vi "chooseSignal.vi"(7 "countIN":dbl, 8 "Direction":string, 9 "signalIN":dbl[](array[numeric]), 10 "chosen?":bool, 11 "Path":string) -> (1 "signalOUT":dbl[](array[numeric]), 6 "countOUT":dbl)   [LabVIEW 2019]
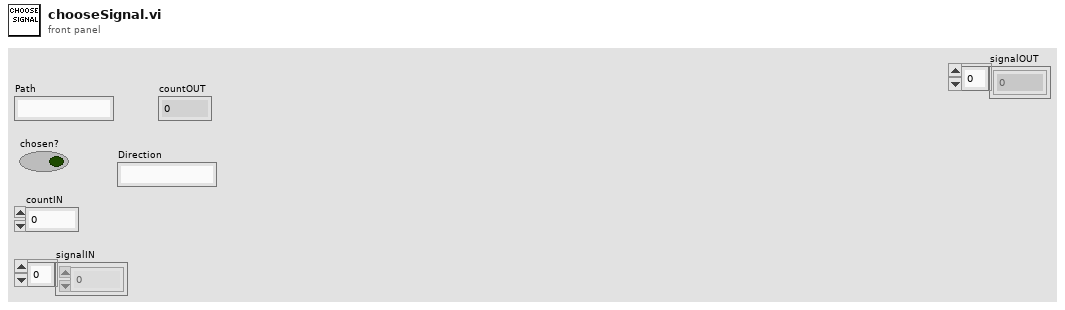
[diagram p1: front panel]
types:
  T1 = enum16{"open", "replace", "create", "open or create", "replace or create", "replace or create with confirmation"}
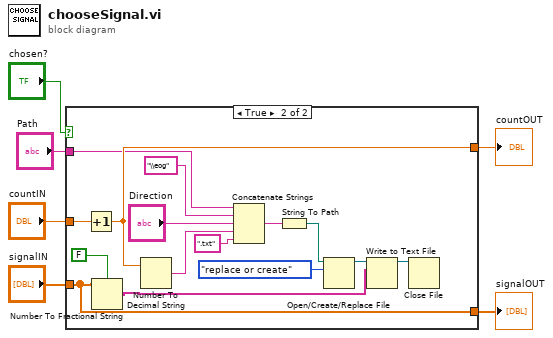
[diagram p0: block diagram]
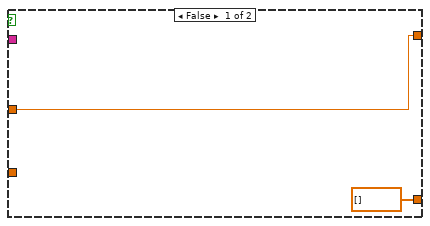
[diagram p2: hidden frame]
diagram:
  n1 = case shown="True" "chosen?" {
    tunnel: "countIN" -> [w8 w23]
    tunnel: [w8 w22] -> w3
    tunnel: [dbl[] [] ("pico -") w10] -> w1
    tunnel: "Path" -> [_ w14]
    tunnel: "signalIN" -> [_ w10]
    frame False {
    }
    frame True {
      n2 = Increment(x=w23) -> (x+1=w22:dbl)
      n3 = Number To Fractional String(use system decimal point (T)=FALSE, number=w10) -> (F-format string=w11:string[])  [unwired: 2 in]
      n4 = Number To Decimal String(number=w22) -> (decimal integer string=w21:string)  [unwired: 1 in]
      n5 = Concatenate Strings(w14, "\\eog" ("string"), "Direction", w21, ".txt" ("string")) -> (w19:string)
      n6 = String To Path(string=w19) -> (path=w18:path)
      n7 = Open/Create/Replace File(file path (use dialog)=w18, operation (0:open)=T1."replace or create") -> (refnum out=w16:refnum<file>)  [unwired: 4 in, 2 out]
      n8 = Write to Text File(file (use dialog)=w16, text=w11) -> (refnum out=w17:refnum<file>)  [unwired: 2 in, 2 out]
      n9 = Close File(refnum=w17) -> ()  [unwired: 1 in, 2 out]
    }
  }
  "countOUT" <- w3
  "signalOUT" <- w1
